vi "AE Upper Off Angle.vi"(9 "Results 2":T1(array[cluster]) {"Normalized Center"."x" format="%#_2g"; "Normalized Center"."y" format="%#_2g"; "Overall Score" format="%#_2g"; "Distance (ft)" format="%#_3g"; "Area Score" format="%#_2g"; "Moment Score" format="%#_2g"; "Aspect Score" format="%#_2g"}, 11 "Port Angle":dbl) -> (2 "x .and. y?":bool, 3 "Port Angle Out":dbl)   [LabVIEW 2025]
uses:
  <vilib>/Rock Robotics/Network Tables/NT Write Number.vi
panel:
  out "Port Distance Out":dbl
  # "Scores"
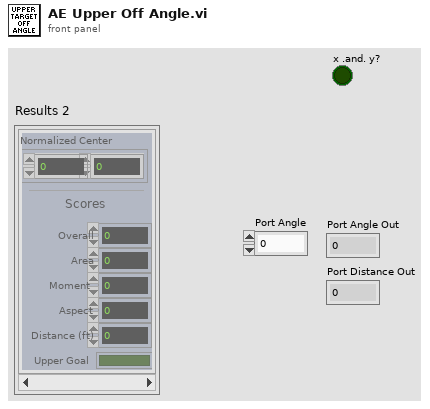
[diagram p1: front panel]
types:
  T1 = cluster{"diameter points":cluster{"first point":cluster{"x":dbl, "y":dbl}, "projected point":cluster{"x":dbl, "y":dbl}}, "Normalized Center":cluster{"x":dbl, "y":dbl}, "Overall Score":dbl, "Area Score":dbl, "Moment Score":dbl, "Aspect Score":dbl, "Distance (ft)":dbl, "Upper Goal":bool}[]
  T2 = cluster{"diameter points":cluster{"first point":cluster{"x":dbl, "y":dbl}, "projected point":cluster{"x":dbl, "y":dbl}}, "Normalized Center":cluster{"x":dbl, "y":dbl}, "Overall Score":dbl, "Area Score":dbl, "Moment Score":dbl, "Aspect Score":dbl, "Distance (ft)":dbl, "Upper Goal":bool}
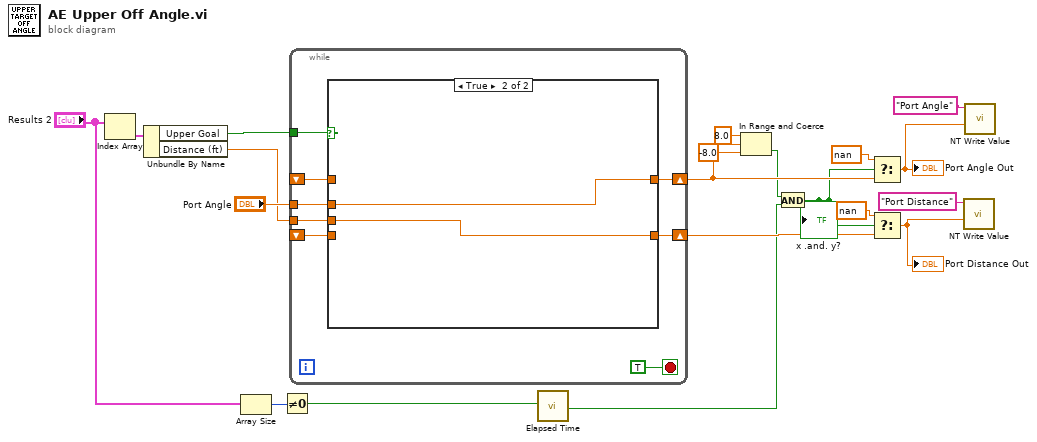
[diagram p0: block diagram]
diagram:
  n1 = Index Array(array="Results 2") -> (element=w19:T2)  [unwired: 1 in]
  n2 = Unbundle By Name(w19) -> ("Upper Goal"=w18:bool, "Distance (ft)"=w10:dbl)
  n3 = Array Size(array="Results 2") -> (size(s)=w16:i32)
  n4 = Not Equal To 0?(x=w16) -> (x != 0?=w14:bool)
  n5 = while {
    tunnel: w18 -> [w28]
    shift-right: [w27] -> w6
    shift-left: _ -> [w25]
    tunnel: "Port Angle" -> [w26]
    shift-right: [w22] -> w8
    shift-left: _ -> [w21]
    tunnel: w10 -> [w23]
    stop <- TRUE stop-if-true
    n6 = case shown="True" w28 {
      tunnel: [w30 w32] -> w27
      tunnel: w26 -> [_ w32]
      tunnel: w25 -> [w30 _]
      tunnel: w23 -> [_ w31]
      tunnel: [w29 w31] -> w22
      tunnel: w21 -> [w29 _]
      frame False {
      }
      frame True {
      }
    }
  }
  n7 = call "Elapsed Time"("Reset"=w14) -> ("Time has Elapsed"=w2:bool)  [unwired: 11 in, 7 out]
  n8 = In Range and Coerce(upper limit=8.0, x=w6, lower limit=-8.0) -> (In Range?=w3:bool)  [unwired: 1 out]
  n9 = And(x=w3, y=w2) -> (x .and. y?=w1:bool)
  "x .and. y?" <- w1
  n10 = Select(t=nan, s=w1, f=w6) -> (s? t:f=w12:dbl)
  "Port Angle Out" <- w12
  n11 = Select(t=nan, s=w1, f=w8) -> (s? t:f=w7:dbl)
  "Port Distance Out" <- w7
  n12 = call-poly <vilib>:"NT Write Value.vi"("value"=w7, "name"="Port Distance" ("Name")) -> ()  [unwired: 9 in, 1 out]
  n13 = call-poly <vilib>:"NT Write Value.vi"("value"=w12, "name"="Port Angle" ("Name")) -> ()  [unwired: 9 in, 1 out]
